vi "NewBegin.vi"(11 "Image Size":T1=enum."160x120") -> (0 "error out":errorcluster)   [LabVIEW 2012]
doc: "Called before other user functions, this VI is expected to open initial I/O refnums, load in file data, and do all program initialization. Notice that the <B>error out</B> terminal is simply used for data flow. Wiring it to other structures or subVIs ensures that this VI runs first."
uses:
  <vilib>/Rock Robotics/WPI/Camera/WPI_CameraImageSize.ctl
  <vilib>/Rock Robotics/WPI/Camera/WPI_CameraWhite Balance Values.ctl
  <vilib>/Rock Robotics/WPI/Camera/WPI_CameraExposure Values.ctl
  <vilib>/Rock Robotics/WPI/Camera/WPI_CameraFrameRate.ctl
  <vilib>/Rock Robotics/WPI/DriverStation/WPI_DriverStationRobotMode2.ctl
  <vilib>/Rock Robotics/WPI/Joystick/WPI_JoystickDeviceEnum.ctl
  <vilib>/Rock Robotics/SystemInterfaces/DIO/FPGA_DIOPWMChannel.ctl
  <vilib>/Rock Robotics/SystemInterfaces/Typedef/FPGA_TypedefAnalogModuleForGyro.ctl
  <vilib>/Rock Robotics/SystemInterfaces/AI/FPGA_AIGyroChannel.ctl
  <vilib>/Rock Robotics/WPI/Solenoid/WPI_SolenoidChannel.ctl
  <vilib>/Rock Robotics/SystemInterfaces/DIO/FPGA_DIORelayChannel.ctl
  <vilib>/Rock Robotics/SystemInterfaces/DIO/FPGA_DIOChannel.ctl
  <vilib>/Rock Robotics/SystemInterfaces/Typedef/FPGA_TypedefDigitalModule.ctl
  <vilib>/Rock Robotics/WPI/Encoder/WPI_EncoderType.ctl
  <vilib>/Rock Robotics/WPI/AnalogChannel/WPI_AnalogChannelDevRef.ctl
  <vilib>/Rock Robotics/SystemInterfaces/Typedef/FPGA_TypedefAnalogModule.ctl
  <vilib>/Rock Robotics/SystemInterfaces/AI/FPGA_AIChannel.ctl
  <vilib>/Rock Robotics/SystemInterfaces/CounterEncoderSourceConvertion/FPGA_CounterEncoderSourceConvertionLVSourceType.ctl
  <vilib>/Rock Robotics/SystemInterfaces/DIO/FPGA_DIODigitalSourceChannel.ctl
  <vilib>/Rock Robotics/SystemInterfaces/AnalogTrigger/FPGA_AnalogTriggerIndex.ctl
  <vilib>/Rock Robotics/SystemInterfaces/AnalogTrigger/FPGA_AnalogTriggerOutType.ctl
  Robot Global Data.vi
  <vilib>/Rock Robotics/WPI/RobotDrive/WPI_RobotDriveOpen2MotorWithTalon.vi
  <vilib>/Rock Robotics/WPI/MotorControl/WPI_MotorControlOpen Talon.vi
  <vilib>/Rock Robotics/WPI/Solenoid/WPI_SolenoidOpenSingle.vi
  <vilib>/Rock Robotics/WPI/Counter/WPI_CounterDigitalInputToDigitalSource.vi
  <vilib>/Rock Robotics/WPI/Counter/WPI_CounterOpen UpDown Mode.vi
  <vilib>/Rock Robotics/WPI/Compressor/WPI_CompressorGetSetRefNum.vi
panel:
  out "error out 2":errorcluster
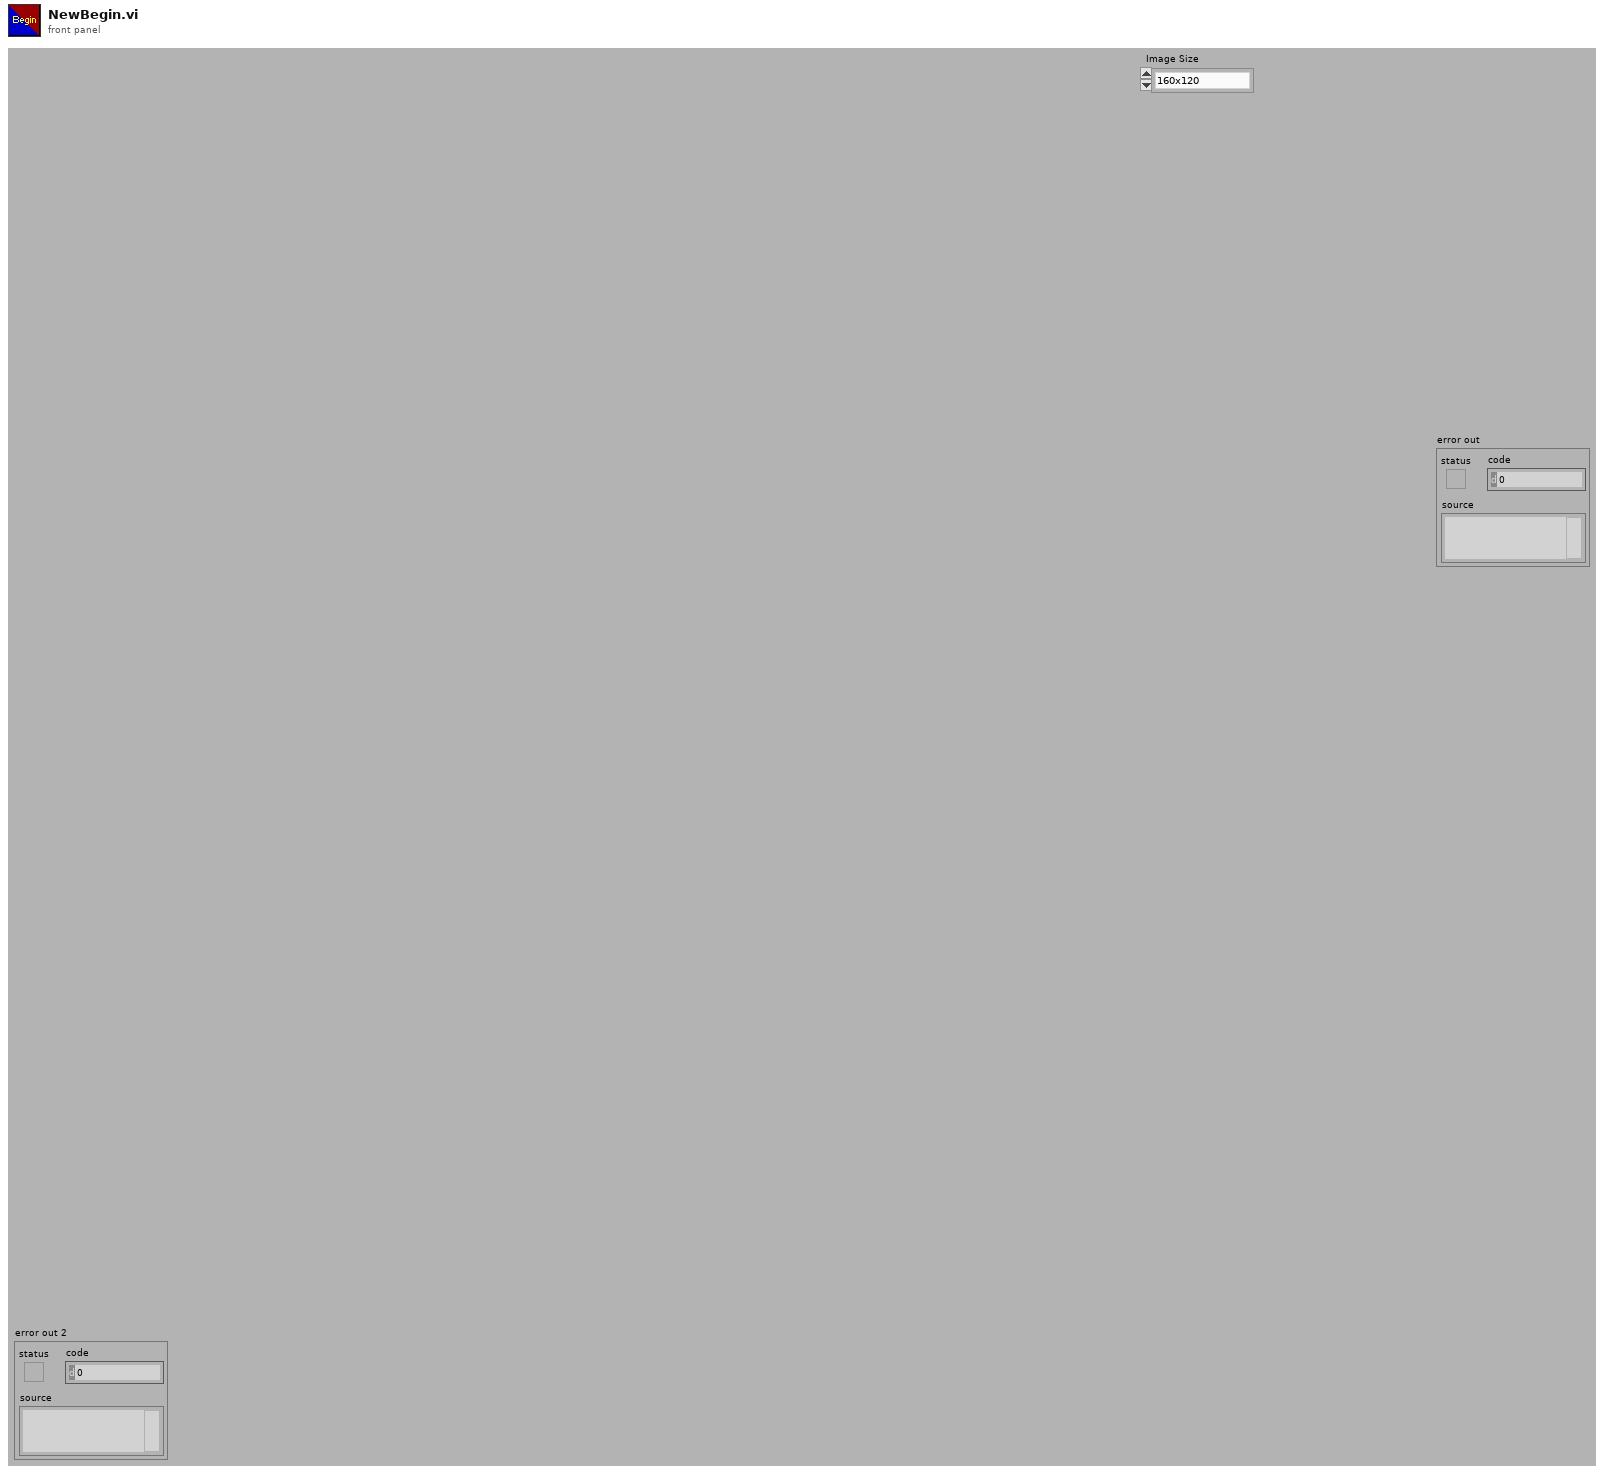
[diagram p1: front panel]
types:
  T1 = typedef "WPI_CameraImageSize.ctl" = enum16{"640x480", "320x240", "160x120"}
  T2 = typedef "FPGA_DIORelayChannel.ctl" = enum8{"Relay 1", "Relay 2", "Relay 3", "Relay 4", "Relay 5", "Relay 6", "Relay 7", "Relay 8", "Invalid"}
  T3 = typedef "FPGA_TypedefDigitalModule.ctl" = enum16{"Digital Module 1", "Digital Module 2"}
  T4 = typedef "WPI_EncoderType.ctl" = enum16{"1x", "2x", "4x"}
  T5 = typedef "FPGA_DIOChannel.ctl" = enum8{"DIO 1", "DIO 2", "DIO 3", "DIO 4", "DIO 5", "DIO 6", "DIO 7", "DIO 8", "DIO 9", "DIO 10", "DIO 11", "DIO 12", "DIO 13", "DIO 14", "Invalid"}
  T6 = typedef "WPI_SolenoidChannel.ctl" = enum8{"Solenoid 1", "Solenoid 2", "Solenoid 3", "Solenoid 4", "Solenoid 5", "Solenoid 6", "Solenoid 7", "Solenoid 8", "Invalid"}
  T7 = typedef "FPGA_DIOPWMChannel.ctl" = enum8{"PWM 1", "PWM 2", "PWM 3", "PWM 4", "PWM 5", "PWM 6", "PWM 7", "PWM 8", "PWM 9", "PWM 10", "Invalid"}
  T8 = enum16{"Rising Edge", "Falling Edge", "Raising & Falling Edge", "Disabled"}
  T9 = typedef "FPGA_CounterEncoderSourceConvertionLVSourceType.ctl" = cluster{"DevStatus":errorcluster, "AnalogTriggerMode?":bool, "DigitalMode":cluster{"Digital Module":T3, "DIO Channel":T10}, "AnalogTriggerMode":cluster{"AnalogTriggerIndex":T11, "OutputType":T12}}
  T10 = typedef "FPGA_DIODigitalSourceChannel.ctl" = enum8{"DIO 1", "DIO 2", "DIO 3", "DIO 4", "DIO 5", "DIO 6", "DIO 7", "DIO 8", "DIO 9", "DIO 10", "DIO 11", "DIO 12", "DIO 13", "DIO 14", "Disabled"}
  T11 = typedef "FPGA_AnalogTriggerIndex.ctl" = enum8{"Trig 0", "Trig 1", "Trig 2", "Trig 3", "Trig 4", "Trig 5", "Trig 6", "Trig 7", "Invalid"}
  T12 = typedef "FPGA_AnalogTriggerOutType.ctl" = enum16{"InWindow", "TriggerState", "Rising", "Falling"}
  T13 = typedef "WPI_AnalogChannelDevRef.ctl" = cluster{"DevStatus":errorcluster, "Analog Module":T14, "Analog Channel":T15}
  T14 = typedef "FPGA_TypedefAnalogModule.ctl" = enum16{"Analog Module 1", "Analog Module 2"}
  T15 = typedef "FPGA_AIChannel.ctl" = enum8{"AI 1", "AI 2", "AI 3", "AI 4", "AI 5", "AI 6", "AI 7", "AI 8", "Invalid"}
  T16 = typedef "FPGA_AIGyroChannel.ctl" = enum8{"AI 1", "AI 2", "Invalid"}
  T17 = typedef "FPGA_TypedefAnalogModuleForGyro.ctl" = enum16{"Analog Module 1"}
  T18 = typedef "WPI_JoystickDeviceEnum.ctl" = enum16{"USB 1", "USB 2", "USB 3", "USB 4", "Kinect 1", "Kinect 2"}
  T19 = typedef "WPI_DriverStationRobotMode2.ctl" = enum16{"Autonomous Disabled", "Autonomous Enabled", "Teleop Disabled", "Teleop Enabled", "Timeout", "Finish", "Test Disabled", "Test Enabled"}
  T20 = typedef "WPI_CameraFrameRate.ctl" = u32
  T21 = typedef "WPI_CameraExposure Values.ctl" = enum16{"Auto", "Flicker-free 50 Hz", "Flicker-free 60 Hz", "Hold current"}
  T22 = typedef "WPI_CameraWhite Balance Values.ctl" = enum16{"Auto", "Fixed indoor", "Fixed outdoor 1", "Fixed outdoor 2", "Fixed fluorescent 1", "Fixed fluorescent 2", "Hold current"}
  T23 = typedef "WPI_SolenoidDevRef.ctl" = cluster{"DevStatus":errorcluster, "Solenoid Module":T24, "Forward Solenoid Channel":T6, "Reverse Solenoid Channel":T6}
  T24 = typedef "FPGA_TypedefSolenoidModule.ctl" = enum16{"Solenoid Module 1", "Solenoid Module 2"}
  T25 = typedef "WPI_DigitalInputDevRef.ctl" = cluster{"DevStatus":errorcluster, "DIO Channel":T5, "Digital Module":T3}
  T26 = typedef "FPGA_AnalogTriggerDevRef.ctl" = cluster{"DevStatus":errorcluster, "AnalogTriggerIndex":T11}
  T27 = typedef "WPI_GyroDevRef.ctl" = cluster{"DevStatus":errorcluster, "Analog Module":T14, "Analog Channel":T15, "Offset":dbl, "Gain (VoltsPerDegree/Second)":dbl}
  T28 = typedef "WPI_CompressorDevRef.ctl" = cluster{"DevStatus":errorcluster, "DigitalInputDevRef":T25, "RelayDevRef":T29}
  T29 = typedef "WPI_RelayDevRef.ctl" = cluster{"DevStatus":errorcluster, "Relay Channel":T2, "Digital Module":T3, "Relay Direction":T30}
  T30 = typedef "WPI_RelayDirection.ctl" = enum16{"Both directions", "Forward only", "Reverse only"}
  T31 = typedef "WPI_CameraDevRef.ctl" = cluster{"Camera Address":string, "CameraStatus":errorcluster, "Acquire Image Notifier":refnum<notifier>}
  T32 = typedef "WPI_JoystickDevRef.ctl" = cluster{"Device":T18}
  T33 = typedef "WPI_CounterDevRef.ctl" = cluster{"DevStatus":errorcluster, "CntIndex":T34}
  T34 = typedef "FPGA_CounterCtrSystemIndex.ctl" = enum8{"Ctr 0", "Ctr 1", "Ctr 2", "Ctr 3", "Ctr 4", "Ctr 5", "Ctr 6", "Ctr 7", "Invalid"}
  T35 = typedef "WPI_MotorControlDeviceRef.ctl" = cluster{"DeviceStatus":errorcluster, "Type":enum16{"PWM", "CAN"}, "PWM":cluster{"Digital Module":T3, "PWM Channel":T7, "DeadBand":T36}, "CAN":cluster{"Device Number":u8, "Control Mode":T37, "Semaphore":T38, "Max Vout":dbl}, "Invert":bool, "TransformRef":T39, "InvTransformRef":T39}
  T36 = typedef "WPI_PWMDeadband.ctl" = cluster{"Name":string, "maxPositivePwm":i32, "minPositivePwm":i32, "centerPwm":i32, "maxNegativePwm":i32, "minNegativePwm":i32, "angularRange":u16}
  T37 = typedef "WPI_CANJaguar_ControlMode.ctl" = enum8{"Percent VBus", "Current", "Speed", "Position", "Voltage"}
  T38 = typedef "Semaphore RefNum" = refnum<k1>
  T39 = typedef "WPI_PWMTransform_ConPane.ctl" = refnum<vi>
  T40 = typedef "WPI_EncoderDevRef.ctl" = cluster{"DevStatus":errorcluster, "EncoderIndex":T41, "CounterIndex":T34, "DistancePerCount":dbl, "Decoding Type":T4}
  T41 = typedef "FPGA_EncoderIdx.ctl" = enum8{"Enc 0", "Enc 1", "Enc 2", "Enc 3", "Invalid"}
  T42 = typedef "WPI_RobotDriveDevRef.ctl" = cluster{"DevStatus":errorcluster, "Motors[]":T35[], "Square Inputs":bool, "Max Output":dbl, "Isochronous":bool}
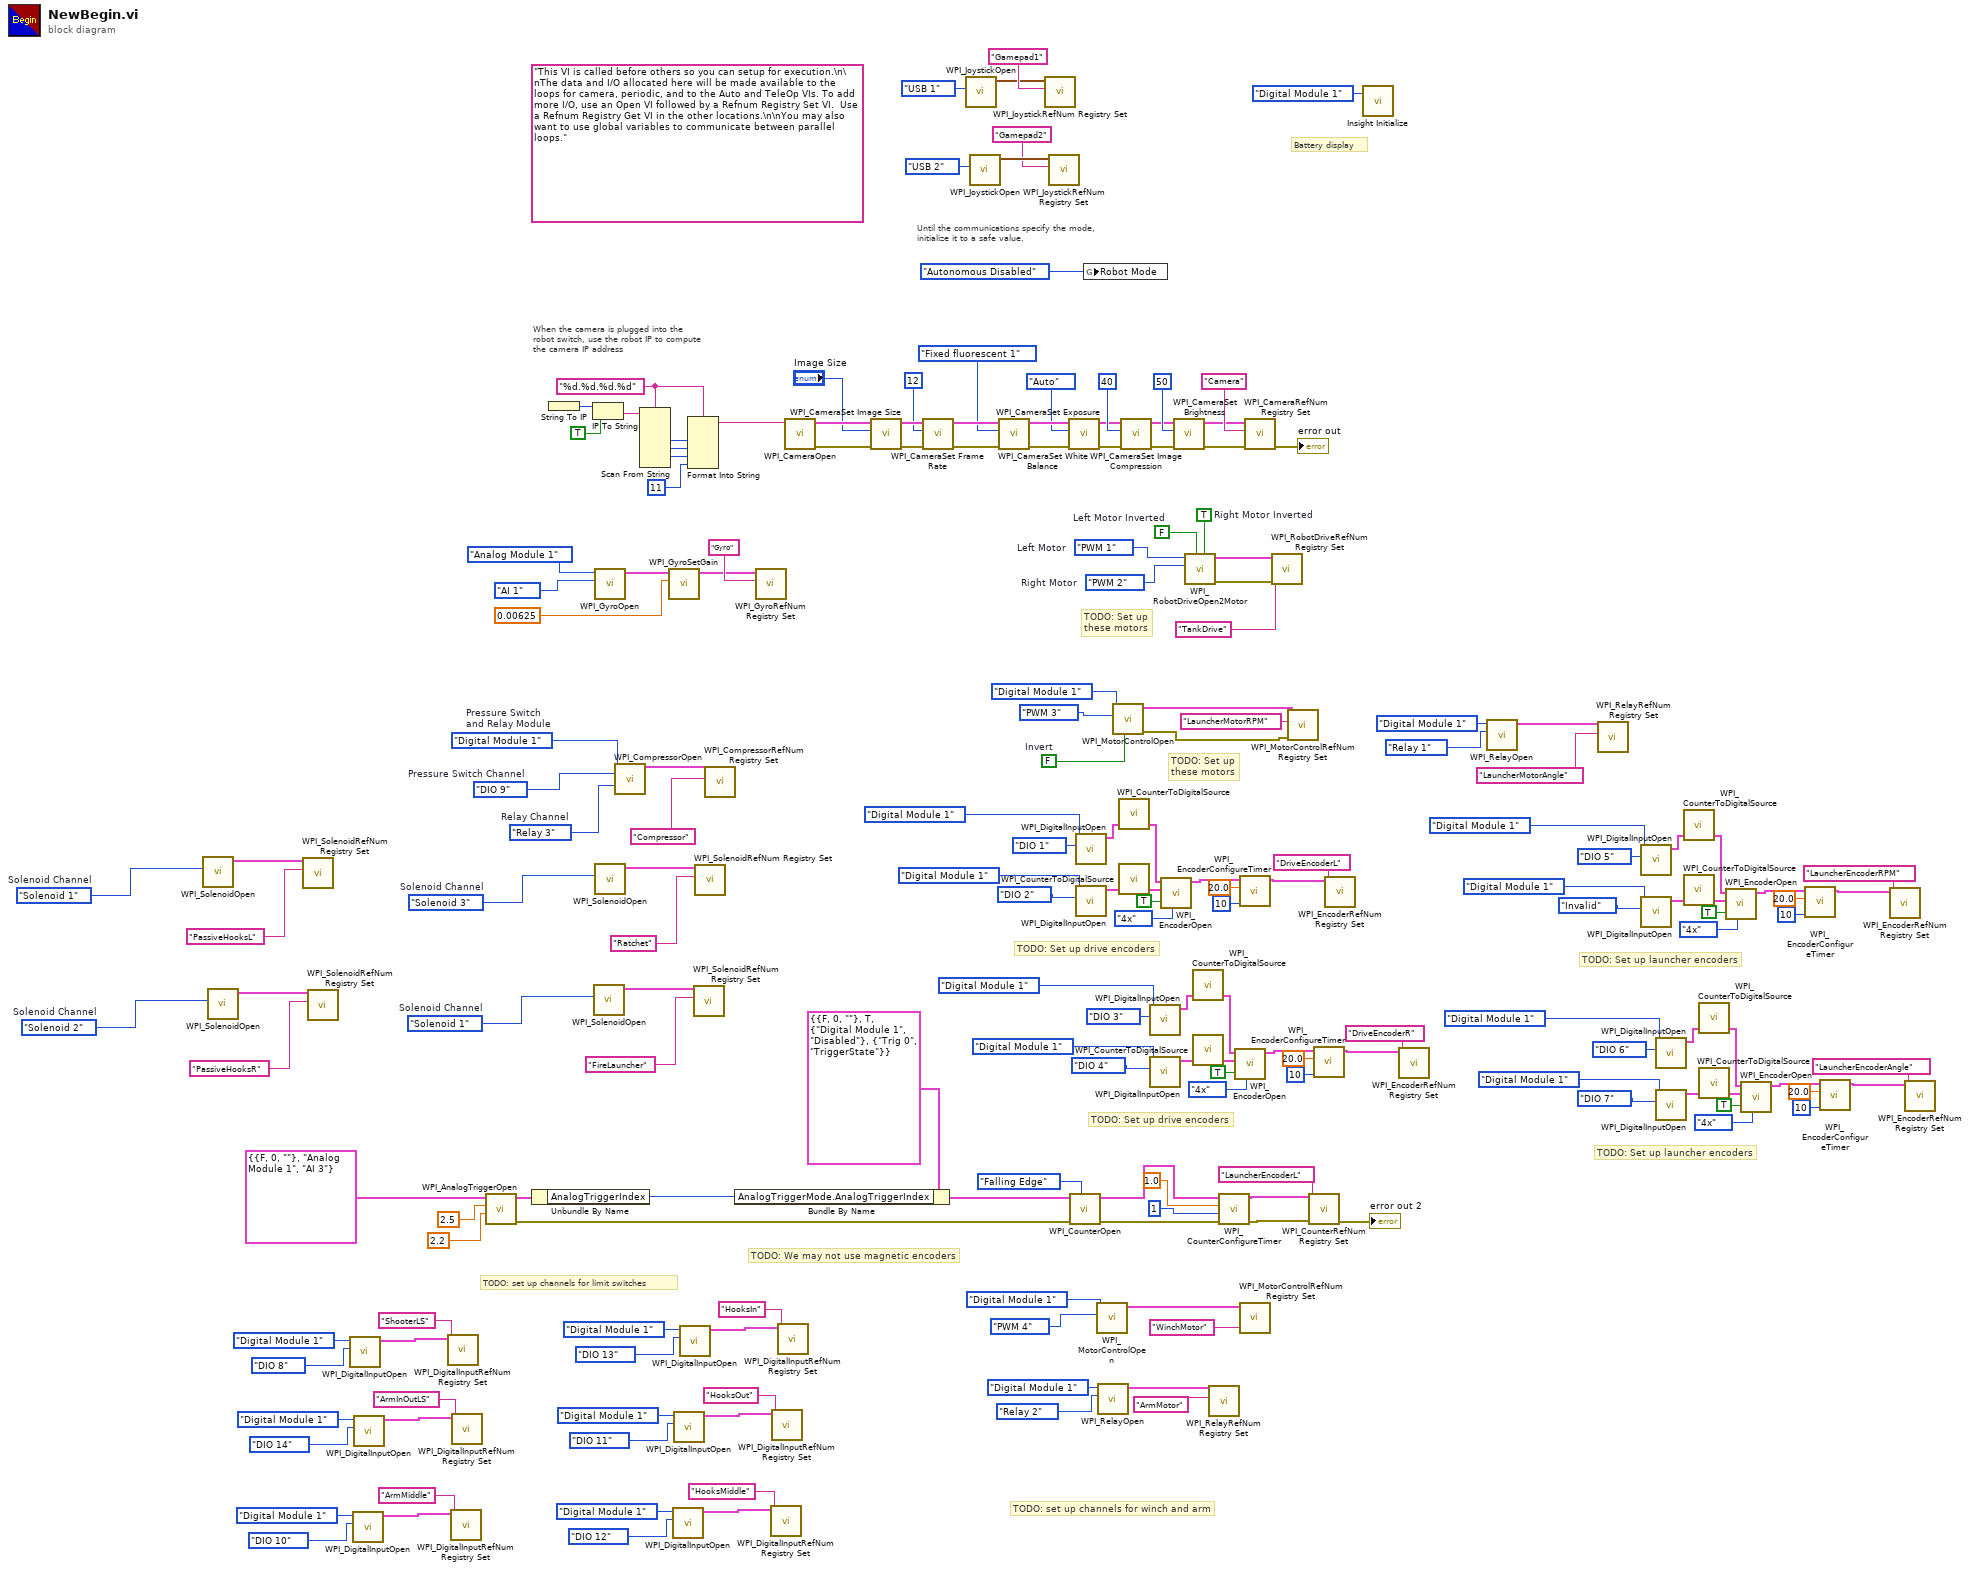
[diagram p0: block diagram]
diagram:
  w41 = WPI_SolenoidChannel."Solenoid 2"  # Solenoid Channel
  w44 = WPI_SolenoidChannel."Solenoid 1"  # Solenoid Channel
  w47 = WPI_SolenoidChannel."Solenoid 1"  # Solenoid Channel
  w129 = FPGA_TypedefDigitalModule."Digital Module 1"  # Pressure Switch and Relay Module
  w131 = FPGA_DIOChannel."DIO 9"  # Pressure Switch Channel
  w130 = FPGA_DIORelayChannel."Relay 3"  # Relay Channel
  w126 = WPI_SolenoidChannel."Solenoid 3"  # Solenoid Channel
  w139 = FALSE  # Invert
  w144 = FPGA_DIOPWMChannel."PWM 2"  # Right Motor
  w145 = FPGA_DIOPWMChannel."PWM 1"  # Left Motor
  w146 = TRUE  # Right Motor Inverted
  w147 = FALSE  # Left Motor Inverted
  w160 = "%d.%d.%d.%d" ("format string")
  (unwired) "This VI is called before others so you can setup for execution.\n\nThe data and I/O allocated here will be made available to the loops for camera, periodic, and to the Auto and TeleOp VIs. To add more I/O, use an Open VI followed by a Refnum Registry Set VI.  Use a Refnum Registry Get VI in the other locations.\n\nYou may also want to use global variables to communicate between parallel loops."
  # "Battery display"
  # "TODO: Set up launcher encoders"
  # "TODO: Set up launcher encoders"
  # "TODO: Set up drive encoders"
  # "TODO: set up channels for winch and arm"
  # "TODO: set up channels for limit switches"
  # "TODO: We may not use magnetic encoders"
  # "TODO: Set up drive encoders"
  # "TODO: Set up\nthese motors"
  # "TODO: Set up\nthese motors"
  # "Until the communications specify the mode,\ninitialize it to a safe value."
  # "When the camera is plugged into the\nrobot switch, use the robot IP to compute\nthe camera IP address"
  n1 = call-poly <vilib>:"WPI_SolenoidOpen.vi"("Solenoid Channel"=w44) -> ("SolenoidDevRef"=w43:T23)  [unwired: 2 in, 8 out]
  n2 = call-poly <vilib>:"WPI_SolenoidOpen.vi"("Solenoid Channel"=w41) -> ("SolenoidDevRef"=w40:T23)  [unwired: 2 in, 8 out]
  n3 = call <vilib>:"WPI_SolenoidRefNum Registry Set.vi"("refnum name"="PassiveHooksL", "SolenoidDevRef"=w43) -> ()  [unwired: 8 in, 2 out]
  n4 = call <vilib>:"WPI_SolenoidRefNum Registry Set.vi"("refnum name"="PassiveHooksR", "SolenoidDevRef"=w40) -> ()  [unwired: 8 in, 2 out]
  n5 = call <vilib>:"WPI_DigitalInputOpen.vi"("DIO Channel"=FPGA_DIOChannel."DIO 8", "Digital Module (Module 1)"=FPGA_TypedefDigitalModule."Digital Module 1") -> ("DigitalInputDevRef"=w71:T25)  [unwired: 8 in, 1 out]
  n6 = call <vilib>:"WPI_DigitalInputOpen.vi"("DIO Channel"=FPGA_DIOChannel."DIO 10", "Digital Module (Module 1)"=FPGA_TypedefDigitalModule."Digital Module 1") -> ("DigitalInputDevRef"=w87:T25)  [unwired: 8 in, 1 out]
  n7 = call <vilib>:"WPI_DigitalInputOpen.vi"("DIO Channel"=FPGA_DIOChannel."DIO 14", "Digital Module (Module 1)"=FPGA_TypedefDigitalModule."Digital Module 1") -> ("DigitalInputDevRef"=w91:T25)  [unwired: 8 in, 1 out]
  n8 = call <vilib>:"WPI_DigitalInputRefNum Registry Set.vi"("refnum name"="ShooterLS", "DigitalInputDevRef"=w71) -> ()  [unwired: 8 in, 2 out]
  n9 = call <vilib>:"WPI_DigitalInputRefNum Registry Set.vi"("refnum name"="ArmMiddle", "DigitalInputDevRef"=w87) -> ()  [unwired: 8 in, 2 out]
  n10 = call <vilib>:"WPI_DigitalInputRefNum Registry Set.vi"("refnum name"="ArmInOutLS", "DigitalInputDevRef"=w91) -> ()  [unwired: 8 in, 2 out]
  n11 = call <vilib>:"WPI_AnalogTriggerOpen.vi"("LowerLimit (v)"=2.2, "UpperLimit (v)"=2.5, "AnalogTriggerSource"=T13 {"DevStatus"={"status"=FALSE, "code"=0, "source"=""}, "Analog Module"=enum."Analog Module 1", "Analog Channel"=enum."AI 3"}) -> ("error out"=w107:errorcluster, "AnalogTriggerDevRef"=w100:T26)  [unwired: 7 in]
  n12 = Unbundle By Name(w100) -> ("AnalogTriggerIndex"=w99:T11)
  n13 = String To IP() -> (0:w167:u32)  [unwired: 1 in]
  n14 = IP To String(1:TRUE ("dot notation? (F)"), 2:w167) -> (0:w165:string)
  n15 = call-poly <vilib>:"WPI_SolenoidOpen.vi"("Solenoid Channel"=w47) -> ("SolenoidDevRef"=w46:T23)  [unwired: 2 in, 8 out]
  n16 = call <vilib>:"WPI_GyroOpen.vi"("Analog Channel"=FPGA_AIGyroChannel."AI 1", "Analog Module (Module 1)"=FPGA_TypedefAnalogModuleForGyro."Analog Module 1") -> ("GyroDevRef"=w134:T27)  [unwired: 7 in, 2 out]
  n17 = call-poly <vilib>:"WPI_SolenoidOpen.vi"("Solenoid Channel"=w126) -> ("SolenoidDevRef"=w125:T23)  [unwired: 2 in, 8 out]
  n18 = call <vilib>:"WPI_CompressorOpen.vi"("Pressure Switch Digital Module (Module 1)"=w129, "Pressure Switch DIO Channel"=w131, "Relay Channel"=w130) -> ("CompressorDevRef"=w128:T28)  [unwired: 2 in, 10 out]
  n19 = Scan From String(format string=w160, input string=w165) -> (output 1=w164:i32, output 2=w163:i32, output 3=w162:i32)  [unwired: 7 in, 3 out]
  n20 = call <vilib>:"WPI_GyroSetGain.vi"("Gain (VoltsPerDegree/Second)"=0.00625, "GyroDevRef"=w134) -> ("GyroDevRef"=w133:T27)  [unwired: 8 in, 1 out]
  n21 = call <vilib>:"WPI_DigitalInputOpen.vi"("DIO Channel"=FPGA_DIOChannel."DIO 12", "Digital Module (Module 1)"=FPGA_TypedefDigitalModule."Digital Module 1") -> ("DigitalInputDevRef"=w75:T25)  [unwired: 8 in, 1 out]
  n22 = call <vilib>:"WPI_DigitalInputOpen.vi"("DIO Channel"=FPGA_DIOChannel."DIO 11", "Digital Module (Module 1)"=FPGA_TypedefDigitalModule."Digital Module 1") -> ("DigitalInputDevRef"=w79:T25)  [unwired: 8 in, 1 out]
  n23 = call <vilib>:"WPI_DigitalInputOpen.vi"("DIO Channel"=FPGA_DIOChannel."DIO 13", "Digital Module (Module 1)"=FPGA_TypedefDigitalModule."Digital Module 1") -> ("DigitalInputDevRef"=w83:T25)  [unwired: 8 in, 1 out]
  n24 = Format Into String(format string=w160, w164, w163, w162, 11 ("Compression")) -> (resulting string=w158:string)  [unwired: 2 in, 1 out]
  n25 = call <vilib>:"WPI_SolenoidRefNum Registry Set.vi"("refnum name"="FireLauncher", "SolenoidDevRef"=w46) -> ()  [unwired: 8 in, 2 out]
  n26 = call <vilib>:"WPI_SolenoidRefNum Registry Set.vi"("refnum name"="Ratchet", "SolenoidDevRef"=w125) -> ()  [unwired: 8 in, 2 out]
  n27 = call <vilib>:"WPI_CompressorRefNum Registry Set.vi"("refnum name"="Compressor", "CompressorDevRef"=w128) -> ()  [unwired: 8 in, 2 out]
  n28 = Bundle By Name(cluster=T9 {"DevStatus"={"status"=FALSE, "code"=0, "source"=""}, "AnalogTriggerMode?"=TRUE, "DigitalMode"={"Digital Module"=enum."Digital Module 1", "DIO Channel"=enum."Disabled"}, "AnalogTriggerMode"={"AnalogTriggerIndex"=enum."Trig 0", "OutputType"=enum."TriggerState"}} ("Source"), "AnalogTriggerMode.AnalogTriggerIndex"=w99) -> (w97:T9)
  n29 = call <vilib>:"WPI_GyroRefNum Registry Set.vi"("refnum name"="Gyro", "GyroDevRef"=w133) -> ()  [unwired: 8 in, 2 out]
  n30 = call <vilib>:"WPI_DigitalInputRefNum Registry Set.vi"("refnum name"="HooksMiddle", "DigitalInputDevRef"=w75) -> ()  [unwired: 8 in, 2 out]
  n31 = call <vilib>:"WPI_DigitalInputRefNum Registry Set.vi"("refnum name"="HooksOut", "DigitalInputDevRef"=w79) -> ()  [unwired: 8 in, 2 out]
  n32 = call <vilib>:"WPI_DigitalInputRefNum Registry Set.vi"("refnum name"="HooksIn", "DigitalInputDevRef"=w83) -> ()  [unwired: 8 in, 2 out]
  n33 = call <vilib>:"WPI_CameraOpen.vi"("Camera Address"=w158) -> ("error out"=w179:errorcluster, "CameraDevRef"=w180:T31)  [unwired: 1 in, 8 out]
  n34 = call <vilib>:"WPI_CameraSet Image Size.vi"("error in (no error)"=w179, "Image Size"="Image Size", "CameraDevRef"=w180) -> ("error out"=w178:errorcluster, "CameraDevRef Out"=w181:T31)  [unwired: 7 out]
  n35 = call <vilib>:"WPI_CameraSet Frame Rate.vi"("error in (no error)"=w178, "Frame Rate (fps)"=T20 12, "CameraDevRef"=w181) -> ("error out"=w177:errorcluster, "CameraDevRef Out"=w183:T31)  [unwired: 7 out]
  n36 = call <vilib>:"WPI_JoystickOpen.vi"("JoystickDevice"=WPI_JoystickDeviceEnum."USB 1") -> ("JoystickDevRef"=w155:T32)  [unwired: 10 in]
  n37 = call <vilib>:"WPI_JoystickOpen.vi"("JoystickDevice"=WPI_JoystickDeviceEnum."USB 2") -> ("JoystickDevRef"=w152:T32)  [unwired: 10 in]
  n38 = call <vilib>:"WPI_CameraSet White Balance.vi"("error in (no error)"=w177, "White Balance"=WPI_CameraWhite_Balance_Values."Fixed fluorescent 1", "CameraDevRef"=w183) -> ("error out"=w176:errorcluster, "CameraDevRef Out"=w182:T31)  [unwired: 7 out]
  n39 = call <vilib>:"WPI_JoystickRefNum Registry Set.vi"("refnum name"="Gamepad1", "JoystickDevRef"=w155) -> ()  [unwired: 8 in, 2 out]
  n40 = call <vilib>:"WPI_JoystickRefNum Registry Set.vi"("refnum name"="Gamepad2", "JoystickDevRef"=w152) -> ()  [unwired: 8 in, 2 out]
  n41 = call <vilib>:"WPI_CameraSet Exposure.vi"("error in (no error)"=w176, "Exposure"=WPI_CameraExposure_Values."Auto", "CameraDevRef"=w182) -> ("error out"=w175:errorcluster, "CameraDevRef Out"=w185:T31)  [unwired: 7 out]
  n42 = call-poly <vilib>:"WPI_CounterOpen.vi"("UpEdge"=T8."Falling Edge" ("UpEdge 1"), "error in (no error)"=w107, "Up Source"=w97) -> ("error out"=w103:errorcluster, "CounterDevRef"=w104:T33)  [unwired: 7 in]
  n43 = call <vilib>:"WPI_DigitalInputOpen.vi"("DIO Channel"=FPGA_DIOChannel."DIO 1", "Digital Module (Module 1)"=FPGA_TypedefDigitalModule."Digital Module 1") -> ("DigitalInputDevRef"=w121:T25)  [unwired: 1 in, 8 out]
  n44 = call <vilib>:"WPI_DigitalInputOpen.vi"("DIO Channel"=FPGA_DIOChannel."DIO 2", "Digital Module (Module 1)"=FPGA_TypedefDigitalModule."Digital Module 1") -> ("DigitalInputDevRef"=w122:T25)  [unwired: 1 in, 8 out]
  n45 = global write "Robot Global Data.vi" "Robot Mode"(WPI_DriverStationRobotMode2."Autonomous Disabled" ("Robot Mode")) -> ()
  n46 = call-poly <vilib>:"WPI_MotorControlOpen.vi"("PWM Channel"=FPGA_DIOPWMChannel."PWM 4", "Digital Module (Module 1)"=FPGA_TypedefDigitalModule."Digital Module 1") -> ("MotorControlDeviceRef"=w65:T35)  [unwired: 8 in, 1 out]
  n47 = call <vilib>:"WPI_RelayOpen.vi"("Relay Channel"=FPGA_DIORelayChannel."Relay 2", "Digital Module (Module 1)"=FPGA_TypedefDigitalModule."Digital Module 1") -> ("RelayDevRef"=w6:T29)  [unwired: 8 in, 1 out]
  n48 = call-poly <vilib>:"WPI_MotorControlOpen.vi"("Invert"=w139, "PWM Channel"=FPGA_DIOPWMChannel."PWM 3", "Digital Module (Module 1)"=FPGA_TypedefDigitalModule."Digital Module 1") -> ("error out"=w138:errorcluster, "MotorControlDeviceRef"=w143:T35)  [unwired: 7 in]
  n49 = call-poly <vilib>:"WPI_CounterToDigitalSource.vi"("DigitalInputDevRef"=w121) -> ("Digital Source"=w120:T9)  [unwired: 6 out]
  n50 = call-poly <vilib>:"WPI_CounterToDigitalSource.vi"("DigitalInputDevRef"=w122) -> ("Digital Source"=w123:T9)  [unwired: 6 out]
  n51 = call <vilib>:"WPI_CameraSet Image Compression.vi"("error in (no error)"=w175, "Compression"=40, "CameraDevRef"=w185) -> ("error out"=w174:errorcluster, "CameraDevRef Out"=w184:T31)  [unwired: 7 out]
  n52 = call <vilib>:"WPI_DigitalInputOpen.vi"("DIO Channel"=FPGA_DIOChannel."DIO 3", "Digital Module (Module 1)"=FPGA_TypedefDigitalModule."Digital Module 1") -> ("DigitalInputDevRef"=w60:T25)  [unwired: 1 in, 8 out]
  n53 = call <vilib>:"WPI_DigitalInputOpen.vi"("DIO Channel"=FPGA_DIOChannel."DIO 4", "Digital Module (Module 1)"=FPGA_TypedefDigitalModule."Digital Module 1") -> ("DigitalInputDevRef"=w61:T25)  [unwired: 1 in, 8 out]
  n54 = call <vilib>:"WPI_EncoderOpen.vi"("Decoding Type"=WPI_EncoderType."4x", "Invert Direction (False)"=TRUE, "BSource"=w123, "ASource"=w120) -> ("EncoderDevRef"=w117:T40)  [unwired: 4 in, 3 out]
  n55 = call <vilib>:"WPI_CameraSet Brightness.vi"("error in (no error)"=w174, "Brightness"=50, "CameraDevRef"=w184) -> ("error out"=w172:errorcluster, "CameraDevRef Out"=w173:T31)  [unwired: 7 out]
  n56 = call-poly <vilib>:"WPI_RobotDriveOpen2Motor.vi"("Right Motor Inverted"=w146, "Left Motor Inverted"=w147, "Right Motor"=w144, "Left Motor"=w145) -> ("error out"=w148:errorcluster, "RobotDriveDevRef"=w150:T42)  [unwired: 6 in]
  n57 = call-poly <vilib>:"WPI_CounterToDigitalSource.vi"("DigitalInputDevRef"=w60) -> ("Digital Source"=w59:T9)  [unwired: 6 out]
  n58 = call-poly <vilib>:"WPI_CounterToDigitalSource.vi"("DigitalInputDevRef"=w61) -> ("Digital Source"=w62:T9)  [unwired: 6 out]
  n59 = call <vilib>:"WPI_RelayRefNum Registry Set.vi"("refnum name"="ArmMotor", "RelayDevRef"=w6) -> ()  [unwired: 8 in, 2 out]
  n60 = call <vilib>:"WPI_CounterConfigureTimer.vi"("error in (no error)"=w103, "Number Samples to Average"=u8 1, "MaxPeriod (sec)"=1.0, "CounterDevRef in"=w104) -> ("error out"=w93:errorcluster, "CounterDevRef out"=w94:T33)  [unwired: 6 in]
  n61 = call <vilib>:"WPI_EncoderOpen.vi"("Decoding Type"=WPI_EncoderType."4x", "Invert Direction (False)"=TRUE, "BSource"=w62, "ASource"=w59) -> ("EncoderDevRef"=w56:T40)  [unwired: 4 in, 3 out]
  n62 = call <vilib>:"WPI_EncoderConfigureTimer.vi"("Number Samples to Average"=u8 10, "Minimum Rate"=20.0, "EncoderDevRef"=w117) -> ("EncoderDevRef"=w114:T40)  [unwired: 1 in, 7 out]
  n63 = call <vilib>:"WPI_MotorControlRefNum Registry Set.vi"("refnum name"="WinchMotor", "MotorControlDevRef"=w65) -> ()  [unwired: 8 in, 2 out]
  n64 = call <vilib>:"WPI_CameraRefNum Registry Set.vi"("error in (no error)"=w172, "refnum name"="Camera", "CameraDevRef"=w173) -> ("error out"=→"error out":errorcluster)  [unwired: 8 out]
  n65 = call <vilib>:"WPI_RobotDriveRefNum Registry Set.vi"("error in (no error)"=w148, "refnum name"="TankDrive", "RobotDriveDevRef"=w150) -> ()  [unwired: 7 in, 2 out]
  n66 = call <vilib>:"WPI_MotorControlRefNum Registry Set.vi"("error in (no error)"=w138, "refnum name"="LauncherMotorRPM", "MotorControlDevRef"=w143) -> ()  [unwired: 7 in, 2 out]
  n67 = call <vilib>:"WPI_CounterRefNum Registry Set.vi"("error in (no error)"=w93, "refnum name"="LauncherEncoderL", "CounterDevRef"=w94) -> ("error out"=→"error out 2":errorcluster)  [unwired: 7 in, 1 out]
  n68 = call <vilib>:"WPI_EncoderConfigureTimer.vi"("Number Samples to Average"=u8 10, "Minimum Rate"=20.0, "EncoderDevRef"=w56) -> ("EncoderDevRef"=w53:T40)  [unwired: 1 in, 7 out]
  n69 = call <vilib>:"WPI_EncoderRefNum Registry Set.vi"("refnum name"="DriveEncoderL", "EncoderDevRef"=w114) -> ()  [unwired: 8 in, 2 out]
  n70 = call "Insight Initialize.vi"("Digital Module"=FPGA_TypedefDigitalModule."Digital Module 1") -> ()  [unwired: 2 in]
  n71 = call <vilib>:"WPI_EncoderRefNum Registry Set.vi"("refnum name"="DriveEncoderR", "EncoderDevRef"=w53) -> ()  [unwired: 8 in, 2 out]
  n72 = call <vilib>:"WPI_RelayOpen.vi"("Relay Channel"=FPGA_DIORelayChannel."Relay 1", "Digital Module (Module 1)"=FPGA_TypedefDigitalModule."Digital Module 1") -> ("RelayDevRef"=w2:T29)  [unwired: 8 in, 1 out]
  n73 = call <vilib>:"WPI_RelayRefNum Registry Set.vi"("refnum name"="LauncherMotorAngle", "RelayDevRef"=w2) -> ()  [unwired: 8 in, 2 out]
  n74 = call <vilib>:"WPI_DigitalInputOpen.vi"("DIO Channel"=FPGA_DIOChannel."DIO 5", "Digital Module (Module 1)"=FPGA_TypedefDigitalModule."Digital Module 1") -> ("DigitalInputDevRef"=w36:T25)  [unwired: 1 in, 8 out]
  n75 = call <vilib>:"WPI_DigitalInputOpen.vi"("DIO Channel"=FPGA_DIOChannel."Invalid", "Digital Module (Module 1)"=FPGA_TypedefDigitalModule."Digital Module 1") -> ("DigitalInputDevRef"=w37:T25)  [unwired: 1 in, 8 out]
  n76 = call <vilib>:"WPI_DigitalInputOpen.vi"("DIO Channel"=FPGA_DIOChannel."DIO 6", "Digital Module (Module 1)"=FPGA_TypedefDigitalModule."Digital Module 1") -> ("DigitalInputDevRef"=w21:T25)  [unwired: 1 in, 8 out]
  n77 = call <vilib>:"WPI_DigitalInputOpen.vi"("DIO Channel"=FPGA_DIOChannel."DIO 7", "Digital Module (Module 1)"=FPGA_TypedefDigitalModule."Digital Module 1") -> ("DigitalInputDevRef"=w22:T25)  [unwired: 1 in, 8 out]
  n78 = call-poly <vilib>:"WPI_CounterToDigitalSource.vi"("DigitalInputDevRef"=w36) -> ("Digital Source"=w35:T9)  [unwired: 6 out]
  n79 = call-poly <vilib>:"WPI_CounterToDigitalSource.vi"("DigitalInputDevRef"=w37) -> ("Digital Source"=w38:T9)  [unwired: 6 out]
  n80 = call-poly <vilib>:"WPI_CounterToDigitalSource.vi"("DigitalInputDevRef"=w21) -> ("Digital Source"=w20:T9)  [unwired: 6 out]
  n81 = call-poly <vilib>:"WPI_CounterToDigitalSource.vi"("DigitalInputDevRef"=w22) -> ("Digital Source"=w23:T9)  [unwired: 6 out]
  n82 = call <vilib>:"WPI_EncoderOpen.vi"("Decoding Type"=WPI_EncoderType."4x", "Invert Direction (False)"=TRUE, "BSource"=w38, "ASource"=w35) -> ("EncoderDevRef"=w32:T40)  [unwired: 4 in, 3 out]
  n83 = call <vilib>:"WPI_EncoderOpen.vi"("Decoding Type"=WPI_EncoderType."4x", "Invert Direction (False)"=TRUE, "BSource"=w23, "ASource"=w20) -> ("EncoderDevRef"=w17:T40)  [unwired: 4 in, 3 out]
  n84 = call <vilib>:"WPI_EncoderConfigureTimer.vi"("Number Samples to Average"=u8 10, "Minimum Rate"=20.0, "EncoderDevRef"=w32) -> ("EncoderDevRef"=w29:T40)  [unwired: 1 in, 7 out]
  n85 = call <vilib>:"WPI_EncoderConfigureTimer.vi"("Number Samples to Average"=u8 10, "Minimum Rate"=20.0, "EncoderDevRef"=w17) -> ("EncoderDevRef"=w14:T40)  [unwired: 1 in, 7 out]
  n86 = call <vilib>:"WPI_EncoderRefNum Registry Set.vi"("refnum name"="LauncherEncoderRPM", "EncoderDevRef"=w29) -> ()  [unwired: 8 in, 2 out]
  n87 = call <vilib>:"WPI_EncoderRefNum Registry Set.vi"("refnum name"="LauncherEncoderAngle", "EncoderDevRef"=w14) -> ()  [unwired: 8 in, 2 out]
